vi "Prototype.vi"() -> ()   [LabVIEW 2014]
uses:
  NetworkStream/NetworkStreamData.ctl
  <vilib>/dex/Stream Element Allocation Mode.ctl
  <vilib>/dex/Flush And Wait Empty Condition.ctl
  NetworkStream/NetworkStream.lvlib
  <resource>/objmgr/ni.dex.rc
panel:
  in  "shared variable refnum in":refnum<k21>="ni.var.psp://localhost/DelayLine/Status"
  in  "Stop":bool
  in  "Play Button":bool
  out "data":i32
  out "Status":string="Ready"
  out "Available Elements for Writing":i32
  in  "millisecond multiple":u32=500
  in  "Abort":bool
  in  "reader url":string="//localhost/DelayLine"
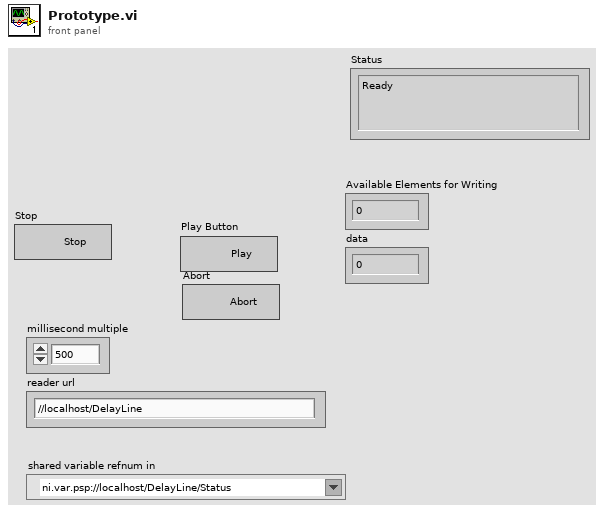
[diagram p1: front panel]
types:
  T1 = typedef "Flush And Wait Empty Condition.ctl" = u8
  T2 = typedef "Stream Element Allocation Mode.ctl" = u32
  T3 = typedef "NetworkStream.lvlib/NetworkStreamData.ctl" = cluster{"Command/Status":string, "Data":variant, "Random Session Hash":u64, "Sequence Number":u64}
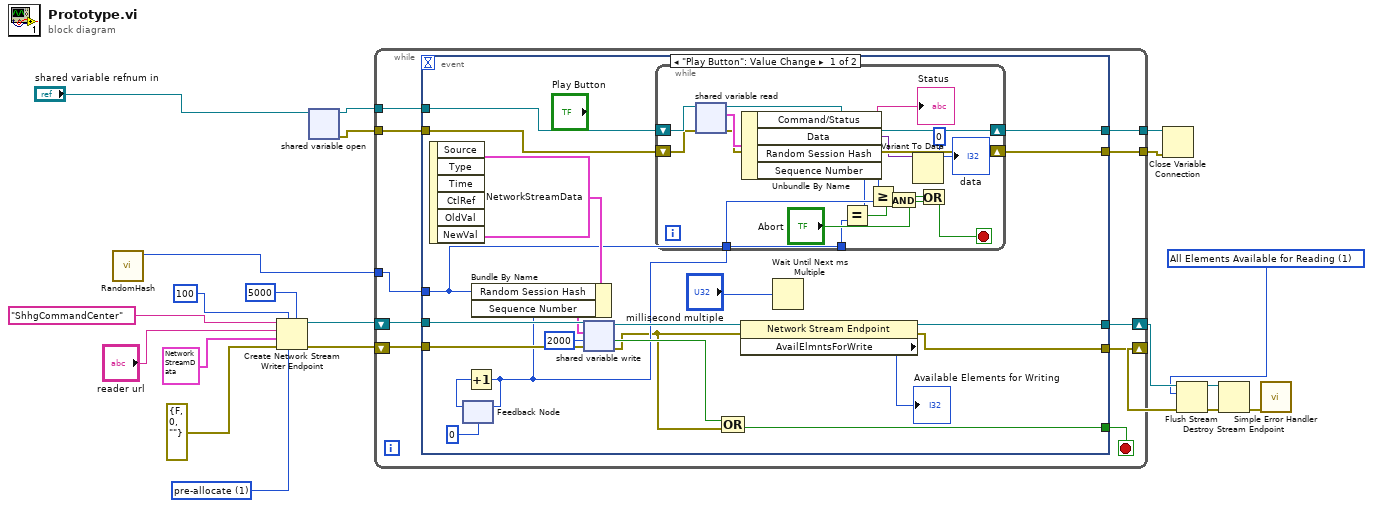
[diagram p0: block diagram]
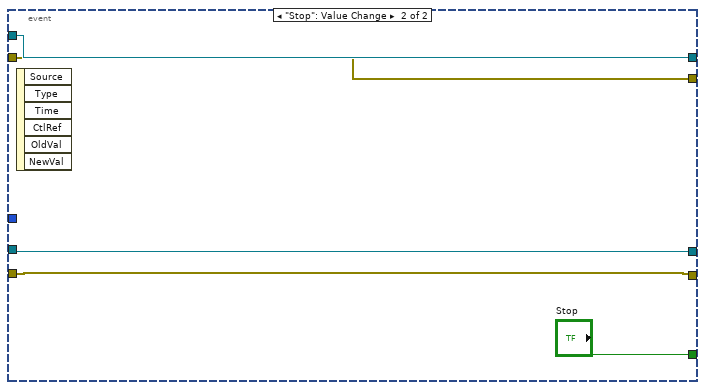
[diagram p2: hidden frame]
diagram:
  w9 = T1 1 items=["All Elements Read From Stream", "All Elements Available for Reading"] ("wait condition")
  w17 = T2 1 items=["allocate as needed", "pre-allocate"] ("element allocation mode")
  n1 = call "RandomHash.vi"() -> ("Numeric Control"=w7:u64)  [unwired: 11 in]
  n2 = Create Network Stream Writer Endpoint(5:5000 ("timeout in ms (-1)"), 6:w17, 7:100 ("writer buffer size"), 8:errorcluster {"status"=FALSE, "code"=0, "source"=""} ("error in (no error)"), 9:T3 {"Command/Status"="", "Data"=variant, "Random Session Hash"=0, "Sequence Number"=0} ("NetworkStreamCluster"), 10:"reader url", 11:"ShhgCommandCenter" ("writer name")) -> (0:w14:errorcluster, 3:w15:refnum<k21>)
  n3 = shared-variable-open("shared variable refnum in") -> (w5:refnum<k21>, w3:errorcluster)  [unwired: 1 in]
  n4 = while {
    shift-right: [w26] -> w13
    shift-left: w15 -> [w31]
    shift-right: [w27] -> w11
    shift-left: w14 -> [w30]
    tunnel: w7 -> [w28]
    tunnel: w5 -> [w25]
    tunnel: [w24] -> w4
    tunnel: w3 -> [w23]
    tunnel: [w22] -> w2
    stop <- w29 stop-if-true
    n5 = event shown="[0] \"Play Button\": Value Change" {
      selector: _ -> [_ _]
      dyn-events: _ -> [_ _]
      timeout: _ -> [_ _]
      tunnel: w31 -> [w52 w73]
      tunnel: w30 -> [w51 w74]
      tunnel: [w47 "Stop"] -> w29
      tunnel: w28 -> [w32 _]
      tunnel: [w41 w74] -> w27
      tunnel: [w40 w73] -> w26
      tunnel: w25 -> [w38 w72]
      tunnel: [w37 w72] -> w24
      tunnel: w23 -> [w36 w71]
      tunnel: [w35 w71] -> w22
      event "Play Button": Value Change {
        n6 = event-data() -> ()  [unwired: 1 in, 6 out]
        n7 = feedback #1(u64 0) -> (w43:u64)
        n8 = Increment(x=w43) -> (x+1=w34:u64)
        n9 = feedback-in #1(w34) -> ()
        n10 = Bundle By Name(cluster=T3 {"Command/Status"="Random Number", "Data"=variant, "Random Session Hash"=0, "Sequence Number"=0} ("data in"), "Random Session Hash"=w32, "Sequence Number"=w34) -> (w48:T3)
        n11 = shared-variable-write(w52, w51, w48, 2000 ("timeout ms (-1)")) -> (w42:refnum<k21>, w33:errorcluster, w46:bool)
        n12 = while {
          shift-right: [w69] -> w37
          shift-left: w38 -> [w70]
          shift-right: [w66] -> w35
          shift-left: w36 -> [w67]
          tunnel: w34 -> [w64]
          tunnel: w32 -> [w53]
          stop <- w62 stop-if-true
          n13 = shared-variable-read(w70, w67) -> (w69:refnum<k21>, w66:errorcluster, w68:T3)
          n14 = Unbundle By Name(w68) -> ("Command/Status"=→"Status":string, "Data"=w59:variant, "Random Session Hash"=w54:u64, "Sequence Number"=w65:u64)
          n15 = Equal?(x=w54, y=w53) -> (x = y?=w55:bool)
          n16 = Greater Or Equal?(x=w65, y=w64) -> (x >= y?=w63:bool)
          n17 = And(x=w63, y=w55) -> (x .and. y?=w56:bool)
          n18 = Variant To Data(type=0, Variant=w59) -> (data=→"data":i32)  [unwired: 1 in, 1 out]
          n19 = Or(x=w56, y="Abort") -> (x .or. y?=w62:bool)
        }
        n20 = Compound Arithmetic op=OR(w46, w33) -> (w47:bool)
        n21 = property class="Network Stream Endpoint"(reference=w42, error in=w33) -> (reference out=w40:refnum<k21>, error out=w41:errorcluster, "AvailElmntsForWrite"=→"Available Elements for Writing":i32)
        n22 = Wait Until Next ms Multiple(millisecond multiple="millisecond multiple") -> ()  [unwired: 1 out]
      }
      event "Stop": Value Change {
        n23 = event-data() -> ()  [unwired: 1 in, 6 out]
      }
    }
  }
  n24 = Close Variable Connection(8:w2, 11:w4) -> ()  [unwired: 1 out]
  n25 = Flush Stream(8:w11, 10:w9, 11:w13) -> (0:w10:errorcluster, 3:w12:refnum<k21>)  [unwired: 1 in, 1 out]
  n26 = Destroy Stream Endpoint(8:w10, 11:w12) -> (0:w8:errorcluster)
  n27 = call <vilib>:"Simple Error Handler.vi"("error in (no error)"=w8) -> ()  [unwired: 4 in, 5 out]
